vi "Audio Capture Example.vi"() -> ()   [LabVIEW 2020]
doc: "Simple example of audio device capture, saving the acquired data to a WAV file."
uses:
  Controls/Audio Device Config.ctl
  Controls/Audio Device Format.ctl
  Controls/Audio Device Info.ctl
  Controls/Audio Device Type.ctl
  Controls/Audio File Info.ctl
  Controls/WAV Codec Specific Info.ctl
  Controls/WAV Container Format.ctl
  Controls/WAV Data Format.ctl
  d37775a1-27ef-4781-ba3e-b38a0bb78134.vi
  7b5afa26-ffc7-4768-ab84-ffe08a27723a.vi
  Private/Result To Error.vi
  d37775a1-27ef-4781-ba3e-b38a0bb78134.vi/6b901882-6109-4f44-aca5-48e1525e5248.vi
  d37775a1-27ef-4781-ba3e-b38a0bb78134.vi/06c0137a-63d3-4e30-982f-115d83a1188c.vi
  Audio Devices/Get Audio Device Configuration.vi
  Private/Audio Device Refnum To Value.vi
  7b5afa26-ffc7-4768-ab84-ffe08a27723a.vi/fba40667-3e21-44fa-934c-95909d78721c.vi
  Private/Audio File Refnum To Value.vi
  d37775a1-27ef-4781-ba3e-b38a0bb78134.vi/06c0137a-63d3-4e30-982f-115d83a1188c.vi/4b7b629c-2e91-4160-9820-a26af8f6e677.vi
  7b5afa26-ffc7-4768-ab84-ffe08a27723a.vi/fba40667-3e21-44fa-934c-95909d78721c.vi/4b7b629c-2e91-4160-9820-a26af8f6e677.vi
  Audio Files/Polymorphic VIs/Open Audio File Write (WAV).vi
  <vilib>/Utility/Data Type/Get Numeric Information.vi
  <vilib>/Utility/error.llb/Error Cluster From Error Code.vi
  G-Audio.lvlib
panel:
  out "error out":errorcluster
  in  "Stop":bool
  out "Waveform":waveform(i16)[](graph)
  # "Instructions:\n1. Run the VI.\n2. Choose a WAV file location to save the captured audio data to.\n3. The VI will begin audio capture and display the data in the waveform graph.\n4. Press Stop to finish audio capture, and save the WAV fle.\n5. Listen to the recorded WAV with Audio Device Playback Example (G-Audio).vi."
  # "G"
  # "-Audio"
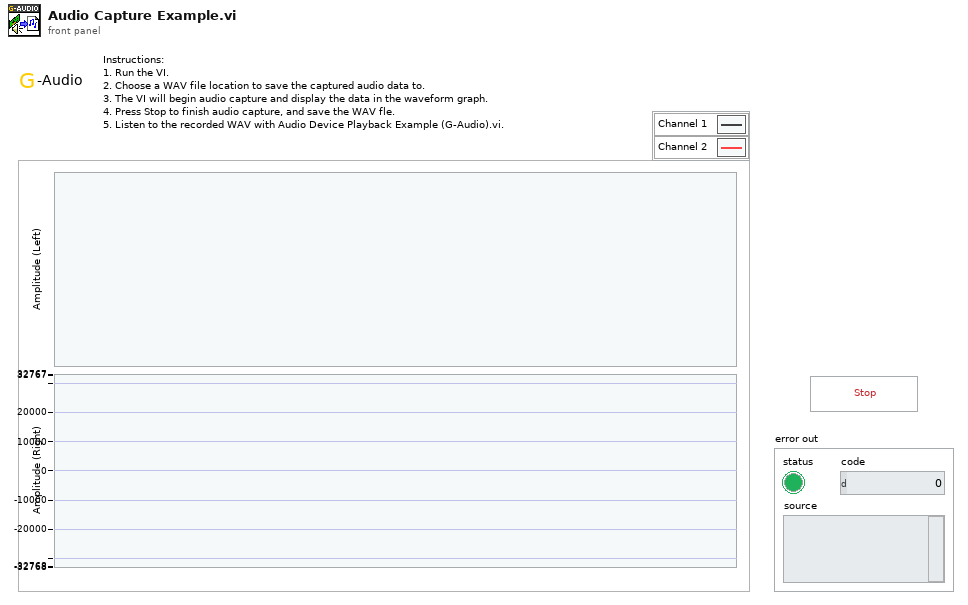
[diagram p1: front panel]
types:
  T1 = typedef "G-Audio.lvlib/Audio Device Type.ctl" = enum16{"(None)", "Playback", "Capture", "Duplex", "Loopback"}
  T2 = typedef "G-Audio.lvlib/WAV Codec Specific Info.ctl" = cluster{"Container Format":T3, "Data Format":T4}
  T3 = typedef "G-Audio.lvlib/WAV Container Format.ctl" = enum32{"RIFF", "Wave64"}
  T4 = typedef "G-Audio.lvlib/WAV Data Format.ctl" = u32
  T5 = typedef "G-Audio.lvlib/Audio File Info.ctl" = cluster{"Sample Rate (Hz)":u32, "Channels":u32, "Bit Depth":u32}
  T6 = typedef "G-Audio.lvlib/Audio Device Info.ctl" = cluster{"Name":string, "ID":u8[], "Device Type":T1, "Default":bool, "Min. Sample Rate (Hz)":u32, "Max. Sample Rate (Hz)":u32, "Min. Channels":u32, "Max. Channels":u32, "Formats":T7[]}
  T7 = typedef "G-Audio.lvlib/Audio Device Format.ctl" = enum16{"Native", "U8", "I16", "I32", "SGL"}
  T8 = typedef "G-Audio.lvlib/Audio Device Config.ctl" = cluster{"Sample Rate (Hz)":u32, "Channels":u32, "Format":T7}
  T9 = typedef "G-Audio.lvlib/Audio File Refnum.ctl" = refnum<file>
  T10 = typedef "G-Audio.lvlib/Audio Device Refnum.ctl" = refnum<file>
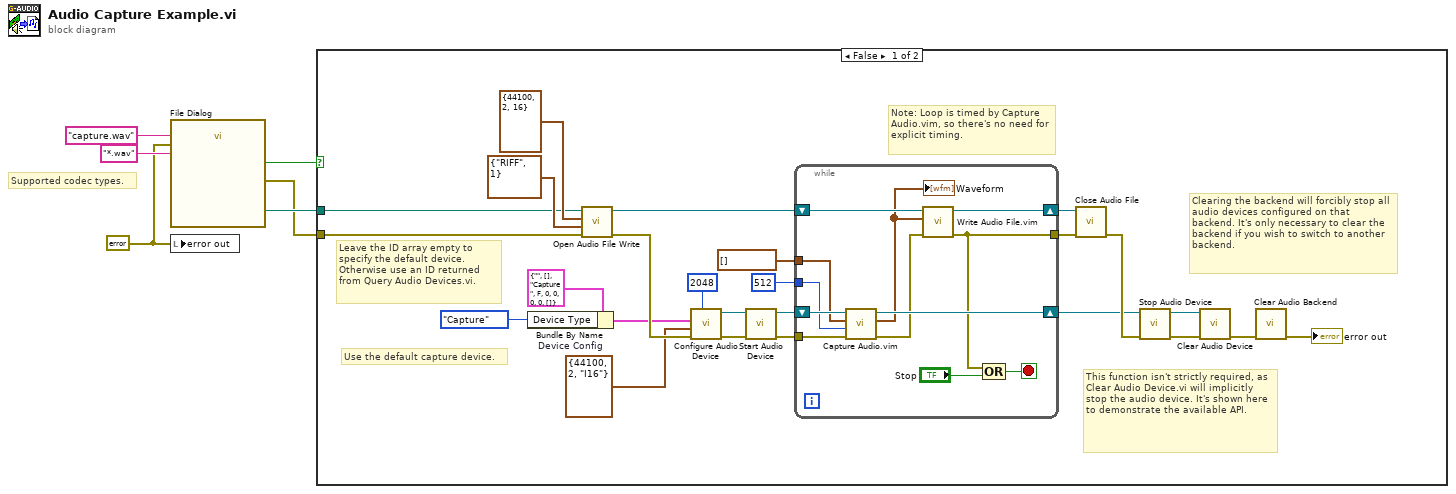
[diagram p0: block diagram]
diagram:
  w2 = errorcluster {"status"=FALSE, "code"=0, "source"=""} ("error out")
  # "Supported codec types."
  n1 = call "File Dialog"("default name"="capture.wav", "error in"=w2, "pattern (all files)"="*.wav") -> ("selected path"=w5:path, "cancelled"=w4:bool, "error out"=w3:errorcluster)  [unwired: 9 in, 1 out]
  n2 = local write "error out"(w2) -> ()
  n3 = case shown="False" w4 {
    tunnel: w5 -> [w11 _]
    tunnel: w3 -> [w14 _]
    frame False {
      w17 = T8 {"Sample Rate (Hz)"=44100, "Channels"=2, "Format"=enum."I16"}  # Device Config
      # "Use the default capture device."
      # "Leave the ID array empty to specify the default device. Otherwise use an ID returned from Query Audio Devices.vi."
      # "This function isn't strictly required, as Clear Audio Device.vi will implicitly stop the audio device. It's shown here to demonstrate the available API."
      # "Clearing the backend will forcibly stop all audio devices configured on that backend. It's only necessary to clear the backend if you wish to switch to another backend."
      # "Note: Loop is timed by Capture Audio.vim, so there's no need for explicit timing."
      n4 = Bundle By Name(cluster=T6 {"Name"="", "ID"=[], "Device Type"=enum."Capture", "Default"=FALSE, "Min. Sample Rate (Hz)"=0, "Max. Sample Rate (Hz)"=0, "Min. Channels"=0, "Max. Channels"=0, "Formats"=[]} ("Audio Device"), "Device Type"=Audio_Device_Type."Capture") -> (w7:T6)
      n5 = call-poly "Open Audio File Write.vi"("error in (no error)"=w14, "Codec Specific Info"=T2 {"Container Format"=enum."RIFF", "Data Format"=1}, "Audio File Info"=T5 {"Sample Rate (Hz)"=44100, "Channels"=2, "Bit Depth"=16}, "Path"=w11) -> ("error out"=w21:errorcluster, "Audio File Refnum"=w23:T9)  [unwired: 6 in]
      n6 = call "Configure Audio Device.vi"("Buffer Size (4096)"=2048 ("number of samples/ch"), "error in (no error)"=w21, "Device Config"=w17, "Audio Device"=w7) -> ("error out"=w20:errorcluster, "Audio Device Refnum"=w19:T10)  [unwired: 4 in, 2 out]
      n7 = call "Start Audio Device.vi"("error in (no error)"=w20, "Audio Device Refnum In"=w19) -> ("error out"=w25:errorcluster, "Audio Device Refnum Out"=w26:T10)  [unwired: 8 in]
      n8 = while {
        shift-right: [w41] -> w31
        shift-left: w23 -> [w43]
        shift-right: [w40] -> w15
        shift-left: w26 -> [w42]
        tunnel: w25 -> [w35]
        tunnel: [w33] -> w29
        tunnel: 512 ("number of samples/ch") -> [w37]
        tunnel: waveform(i16)[] [] -> [w36]
        stop <- w39 stop-if-true
        n9 = call "Capture Audio.vim"("error in (no error)"=w35, "Samples To Read"=w37, "Data Format"=w36, "Audio Device Refnum In"=w42) -> ("error out"=w34:errorcluster, "Audio Data"=w32:waveform(i16)[], "Audio Device Refnum Out"=w40:T10)  [unwired: 5 in]
        "Waveform" <- w32
        n10 = call "Write Audio File.vim"("error in (no error)"=w34, "Audio Data"=w32, "Audio File Refnum In"=w43) -> ("error out"=w33:errorcluster, "Audio File Refnum Out"=w41:T9)  [unwired: 7 in]
        n11 = Compound Arithmetic op=OR(w33, "Stop") -> (w39:bool)
      }
      n12 = call "Close Audio File.vi"("error in (no error)"=w29, "Audio File Refnum In"=w31) -> ("error out"=w28:errorcluster)  [unwired: 9 in]
      n13 = call "Stop Audio Device.vi"("error in (no error)"=w28, "Audio Device Refnum In"=w15) -> ("error out"=w27:errorcluster, "Audio Device Refnum Out"=w30:T10)  [unwired: 8 in]
      n14 = call "Clear Audio Device.vi"("error in (no error)"=w27, "Audio Device Refnum In"=w30) -> ("error out"=w24:errorcluster)  [unwired: 9 in]
      n15 = call "Clear Audio Backend.vi"("error in (no error)"=w24) -> ("error out"=→"error out":errorcluster)  [unwired: 10 in]
    }
    frame True {
    }
  }
